vi "Set Chess.vi"(2 "Pic out":bool, 3 "Move Array":i32[](array[numeric]), 4 "Chess Array":i32[][](array[numeric])=[[140, 130, 120, 110, 100, 111, 121, 131, 141], [-1, -1, -1, -1, -1, -1, -1, -1, -1], [-1, 150, -1, -1, -1, -1, -1, 151, -1], [160, -1, 161, -1, 162, -1, 163, -1, 164], [-1, -1, -1, -1, -1, -1, -1, -1, -1], [-1, -1, -1, -1, -1, -1, -1, -1, -1], [260, -1, 261, -1, 262, -1, 263, -1, 264], [-1, 250, -1, -1, -1, -1, -1, 251, -1], [-1, -1, -1, -1, -1, -1, -1, -1, -1], [240, 230, 220, 210, 200, 211, 221, 231, 241]]) -> (0 "Chess Array Output":i32[][](array[numeric])=[[140, 130, 120, 110, 100, 111, 121, 131, 141], [-1, -1, -1, -1, -1, -1, -1, -1, -1], [-1, 150, -1, -1, -1, -1, -1, 151, -1], [160, -1, 161, -1, 162, -1, 163, -1, 164], [-1, -1, -1, -1, -1, -1, -1, -1, -1], [-1, -1, -1, -1, -1, -1, -1, -1, -1], [260, -1, 261, -1, 262, -1, 263, -1, 264], [-1, 250, -1, -1, -1, -1, -1, 251, -1], [-1, -1, -1, -1, -1, -1, -1, -1, -1], [240, 230, 220, 210, 200, 211, 221, 231, 241]], 1 "Chess":picture)   [LabVIEW 2009]
panel:
  in  "Blank":picture
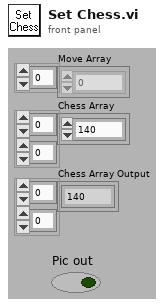
[diagram p1: front panel]
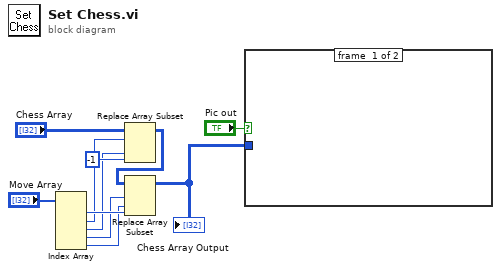
[diagram p0: block diagram]
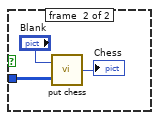
[diagram p2: hidden frame]
diagram:
  n1 = Index Array(array="Move Array") -> (element #1=w8:i32, element #2=w7:i32, element #3=w6:i32, element #4=w5:i32, element #5=w4:i32)  [unwired: 5 in]
  n2 = Replace Array Subset(array="Chess Array", new element=-1 ("New Element/Subarray"), index (row)=w7, index (col)=w6) -> (w10:i32[][])
  n3 = Replace Array Subset(array=w10, new element=w8, index (row)=w5, index (col)=w4) -> (w2:i32[][])
  "Chess Array Output" <- w2
  n4 = case shown="False" "Pic out" {
    tunnel: w2 -> [_ w13]
    frame #0 {
    }
    frame #1 {
      n5 = call "put chess.vi"("Chess Array"=w13, "In Pic"="Blank") -> ("Out Pic"=→"Chess":picture)
    }
  }
